vi "OE2052_RS232_Query Data.vi"(0 "VISA resource name":refnum<visa-resource-name>, 11 "Error in (no error)":errorcluster caption="error out（no error）") -> (4 "VISA resource  out":refnum<visa-resource-name>, 6 "Data Array":dbl[](array[numeric]), 8 "Parameter Values":T1, 10 "Output String":string, 15 "Error out":errorcluster caption="error out")   [LabVIEW 2011]
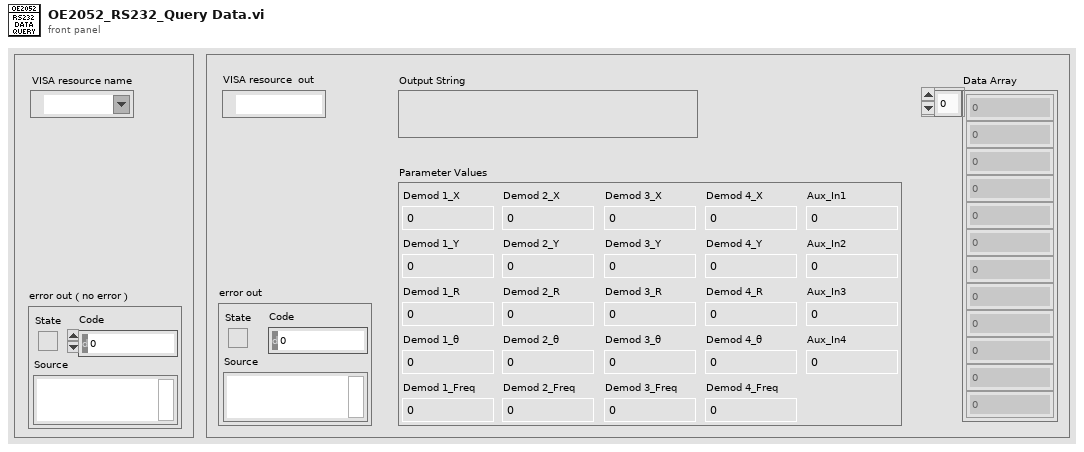
[diagram p1: front panel]
types:
  T1 = cluster{"Demod 1_X":dbl, "Demod 1_Y":dbl, "Demod 1_R":dbl, "Demod 1_θ":dbl, "Demod 1_Freq":dbl, "Demod 2_X":dbl, "Demod 2_Y":dbl, "Demod 2_R":dbl, "Demod 2_θ":dbl, "Demod 2_Freq":dbl, "Demod 3_X":dbl, "Demod 3_Y":dbl, "Demod 3_R":dbl, "Demod 3_θ":dbl, "Demod 3_Freq":dbl, "Demod 4_X":dbl, "Demod 4_Y":dbl, "Demod 4_R":dbl, "Demod 4_θ":dbl, "Demod 4_Freq":dbl, "Aux_In1":dbl, "Aux_In2":dbl, "Aux_In3":dbl, "Aux_In4":dbl}
  T2 = cluster{dbl, dbl, dbl, dbl, dbl, dbl, dbl, dbl, dbl, dbl, dbl, dbl, dbl, dbl, dbl, dbl, dbl, dbl, dbl, dbl, dbl, dbl, dbl, dbl}
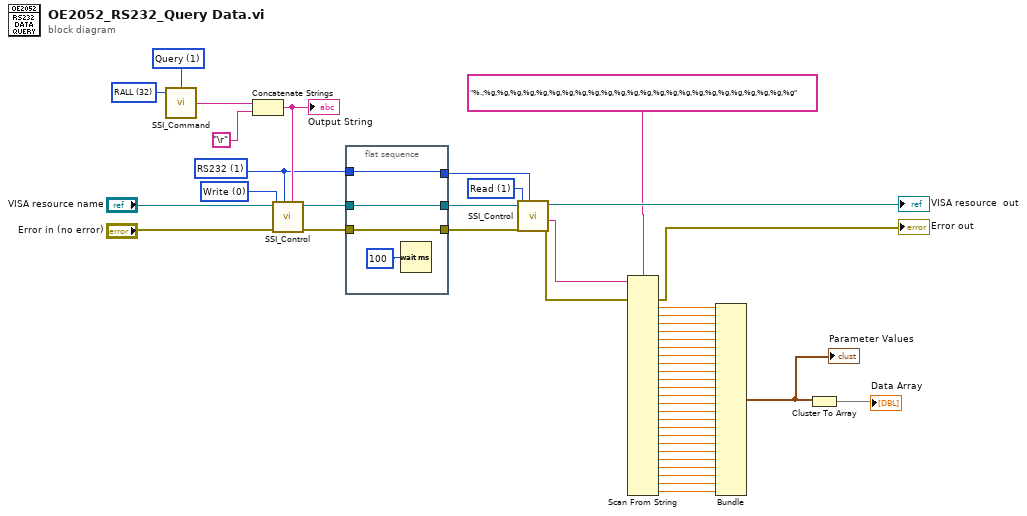
[diagram p0: block diagram]
diagram:
  w32 = u16 1 items=["USB"=0, "RS232"=1, "Ethernet"=3] ("Remote Mode")
  w34 = u16 32 items=["ISRC", "IGND", "ICPL", "ILIN", "PHAS", "FMOD", "RSLP", "FREQ", "SWPT", "SLLM", "SULM", "SSLL", "SSLG", "STLM", "SWRM", "IRNG", "SENS", "RMOD", "OFLT", "OFSL", "SYNC", "DMOD", "HARM", "DARB", "SWVT", "SLVL", "SVLL", "SVUL", "SVSL", "SVSG", "SVTM", "SVRM", "RALL", "SNAP", "OUTP", "OAUX", "COUT", "CAUX", "COFP", "CEXP", "FPOP", "OEXP", "*IDN", "*RST", "OVLD", "INOV", "GNOV", "*PLL", "SSET", "RSET", "AGAN", "APHS", "ARSV", "ASCL", "EQCD", "EQCS", "SPED", "SRAT", "SLEN", "SSLE", "STRG", "SPRM", "STRD", "PAUS", "RSET", "SPTS", "TRCA", "TEMP", "RSTU", "INHZ", "DEQU", "SADD", "ARNG", "CSPE", "ISRCD", "IGNDD", "ICPLD", "ILIND", "PHASD", "FMODD", "RSLPD", "FREQD", "SWPTD", "SLLMD", "SULMD", "SSLLD", "SSLGD", "STLMD", "SWRMD", "SENSD", "RMODD", "OFLTD", "OFSLD", "SYNCD", "HARMD", "EQCDD", "EQCSD", "SNAPD", "OUTPD", "SWVTD", "SLVLD", "SVLLD", "SVULD", "SVSLD", "SVSGD", "SVTMD", "SVRMD", "SVDCD", "ARSVD", "AGAND", "APHSD", "ASCLD", "FPOPD", "CAUXD", "OEXPD", "SPEDD", "SRATD", "SLEND", "SSLED", "STRGD", "SPRMD", "STRDD", "PAUSD", "RESTD", "SPTSD", "TRCAD", "*IDND", "*RSTD", "INOVD", "GNOVD", "*PLLD", "SSETD", "RSETD", "RALLD"] ("Command Type")
  w31 = u16 1 items=["Set", "Query"] ("Opera")
  w38 = u16 1 items=["Write", "Read"] ("Control")
  w43 = u16 0 items=["Write", "Read"] ("Control")
  n1 = call "SSI_Command.vi"("Opera"=w31, "Command Type"=w34) -> ("Output string"=w33:string)  [unwired: 2 in]
  n2 = Concatenate Strings(w33, "\r") -> (w35:string)
  "Output String" <- w35
  n3 = call "SSI_Control.vi"("Write Buffer"=w35, "Remote Mode"=w32, "Error in (no error)"="Error in (no error)", "Control"=w43, "VISA resource name"="VISA resource name") -> ("Error out"=w41:errorcluster, "VISA resource  out"=w42:refnum<visa-resource-name>)  [unwired: 3 in, 2 out]
  n4 = flat-sequence {
    tunnel: w42 -> [w50]
    tunnel: w41 -> [w49]
    tunnel: [w50] -> w40
    tunnel: [w49] -> w39
    tunnel: [w47] -> w37
    tunnel: w32 -> [w47]
    frame #0 {
      n5 = Wait (ms)(milliseconds to wait=u32 100 ("等待时间（毫秒）")) -> ()  [unwired: 1 out]
    }
  }
  n6 = call "SSI_Control.vi"("Remote Mode"=w37, "Error in (no error)"=w39, "Control"=w38, "VISA resource name"=w40) -> ("Error out"=w4:errorcluster, "Read Buffer"=w5:string, "VISA resource  out"=→"VISA resource  out":refnum<visa-resource-name>)  [unwired: 4 in, 1 out]
  n7 = Scan From String(format string="%.;%g,%g,%g,%g,%g,%g,%g,%g,%g,%g,%g,%g,%g,%g,%g,%g,%g,%g,%g,%g,%g,%g,%g,%g" ("格式字符串"), input string=w5, error in=w4) -> (error out=→"Error out":errorcluster, output 1=w30:dbl, output 2=w29:dbl, output 3=w28:dbl, output 4=w27:dbl, output 5=w26:dbl, output 6=w25:dbl, output 7=w24:dbl, output 8=w23:dbl, output 9=w22:dbl, output 10=w21:dbl, output 11=w20:dbl, output 12=w19:dbl, output 13=w18:dbl, output 14=w17:dbl, output 15=w16:dbl, output 16=w15:dbl, output 17=w14:dbl, output 18=w13:dbl, output 19=w12:dbl, output 20=w7:dbl, output 21=w8:dbl, output 22=w9:dbl, output 23=w10:dbl, output 24=w11:dbl)  [unwired: 25 in, 2 out]
  n8 = Bundle(w30, w29, w28, w27, w26, w25, w24, w23, w22, w21, w20, w19, w18, w17, w16, w15, w14, w13, w12, w7, w8, w9, w10, w11) -> (w2:T2)  [unwired: 1 in]
  "Parameter Values" <- w2
  n9 = Cluster To Array(cluster=w2) -> (array=→"Data Array":dbl[])
